vi "request.To JSON String.vi"(8 "error in (no error)":errorcluster, 11 "Request in":refnum<class "Request.lvclass">) -> (0 "error out":errorcluster, 2 "JSON String":string, 3 "Request out":refnum<class "Request.lvclass">)   [LabVIEW 2017, in "Request.lvclass"]
uses:
  Request.lvclass
  <vilib>/National Instruments/Variant JSON API/Variant JSON API.lvlib
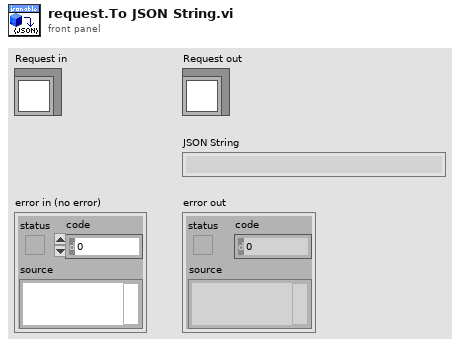
[diagram p1: front panel]
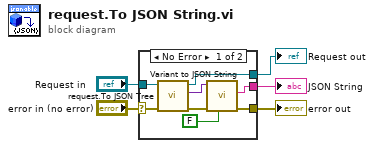
[diagram p0: block diagram]
diagram:
  n1 = case shown="No Error" "error in (no error)" {
    selector: "error in (no error)" -> [w12 w15]
    tunnel: [w8 w15] -> w4
    tunnel: [w11 w14] -> w2
    tunnel: "Request in" -> [w13 w14]
    tunnel: [w9 _] -> w1
    frame No Error {
      n2 = call "request.To JSON Tree.vi"("error in (no error)"=w12, "Request in"=w13) -> ("error out"=w7:errorcluster, "JSON Value out"=w10:variant, "Request out"=w11:refnum<class "Request.lvclass">)  [unwired: 7 in]
      n3 = call <vilib>:"Variant to JSON String.vi"("pretty print? (F)"=FALSE ("pretty print? (T)"), "error in (no error)"=w7, "Variant in"=w10) -> ("error out"=w8:errorcluster, "String"=w9:string)  [unwired: 6 in, 1 out]
    }
    frame Error {
    }
  }
  "error out" <- w4
  "Request out" <- w2
  "JSON String" <- w1
